vi "Concat Stream Data.vi"(8 "error in (no error)":errorcluster, 11 "remaining elements":cluster{"Stream/Aquire Data":dbl[][]}[](array[cluster])) -> (0 "error out":errorcluster, 3 "Stream/Aquire Data":dbl[][](array[numeric]))   [LabVIEW 2024]
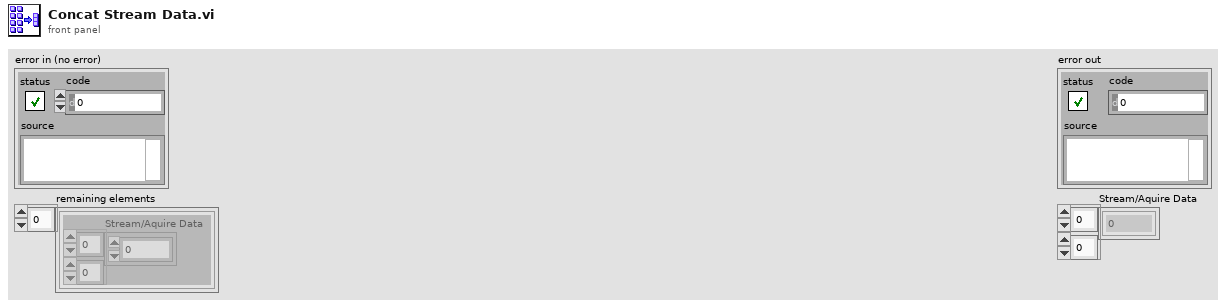
[diagram p1: front panel]
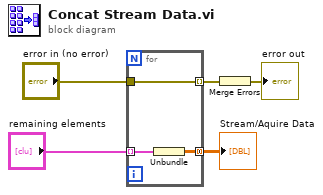
[diagram p0: block diagram]
diagram:
  n1 = for {
    tunnel: [w8] -> w1 mode=indexing
    tunnel: "error in (no error)" -> [w8]
    tunnel: "remaining elements" -> [w7] mode=indexing
    tunnel: [w6] -> w2 mode=concatenating
    n2 = Unbundle(w7) -> ("Stream/Aquire Data"=w6:dbl[][])
  }
  "Stream/Aquire Data" <- w2
  n3 = Merge Errors(w1) -> (→"error out":errorcluster)
